vi "Initialize.vi"(8 "error in":errorcluster, 11 "Ballard ARINC-429 shared resources in":refnum<class "Ballard ARINC-429 Shared Resources.lvclass">) -> (0 "error out":errorcluster, 3 "Ballard ARINC-429 shared resources out":refnum<class "Ballard ARINC-429 Shared Resources.lvclass">)   [LabVIEW 2020, in "Ballard ARINC 429 Engine.lvlib" / "Implementation.lvlib" / "Ballard ARINC-429 Shared Resources.lvclass"]
uses:
  Ballard ARINC-429 Shared Resources.lvclass
  Ballard ARINC-429 Shared Resources.lvclass/Ballard ARINC-429 Shared Resources.ctl
  Custom Device/Custom Device.lvlib
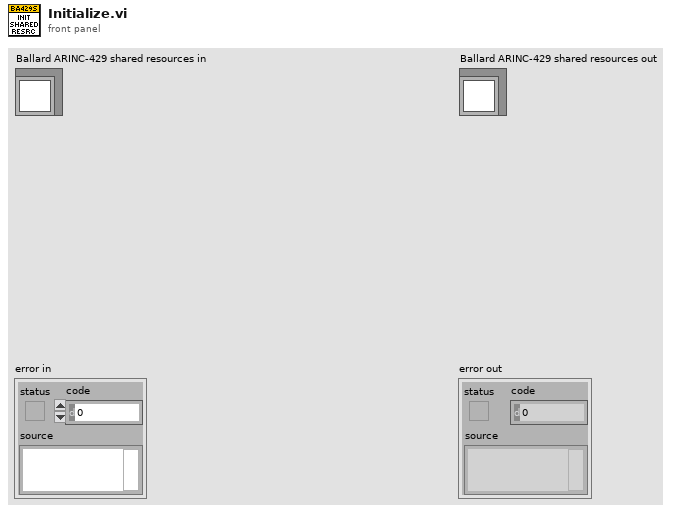
[diagram p1: front panel]
types:
  T1 = typedef "Device Parameters.ctl" = cluster{"initialization method":T2, "card number":i32, "PXI slot number":i32, "core number":i32}
  T2 = typedef "Initialization Method.ctl" = enum16{"PXI Slot Number", "Card Number"}
  T3 = typedef "Ballard ARINC 429 Engine.lvlib/Custom Device.lvlib/Hardware Handles.ctl" = cluster{"core handle":u64, "core reader handle":u64, "channel handles":u64[]}
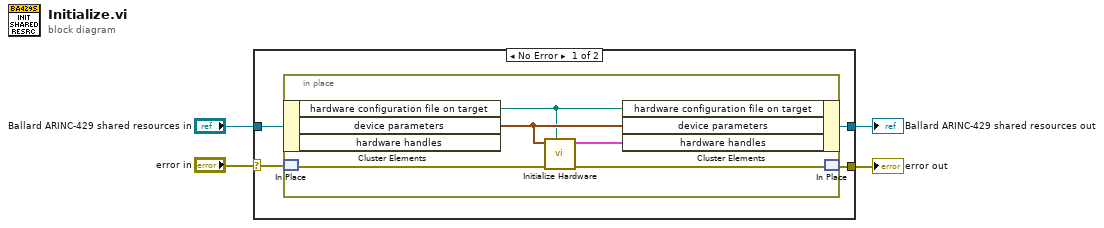
[diagram p0: block diagram]
diagram:
  n1 = case shown="No Error" "error in" {
    selector: "error in" -> [w8 w14]
    tunnel: "Ballard ARINC-429 shared resources in" -> [w6 w15]
    tunnel: [w7 w14] -> w2
    tunnel: [w5 w15] -> w1
    frame No Error {
      n2 = in-place {
        n3 = in-place-cluster #1(w6) -> ("hardware configuration file on target"=w9:path, "device parameters"=w10:T1)  [unwired: 1 out]
        n4 = in-place-match #2(w8) -> (w13:errorcluster)
        n5 = call "Initialize Hardware.vi"("RT config file"=w9, "error in"=w13, "device parameters"=w10) -> ("error out"=w12:errorcluster, "RT handles"=w11:T3)  [unwired: 6 in, 1 out]
        n6 = in-place-cluster #1("hardware configuration file on target"=w9, "device parameters"=w10, "hardware handles"=w11) -> (w5:refnum<class "Ballard ARINC-429 Shared Resources.lvclass">)
        n7 = in-place-match #2(w12) -> (w7:errorcluster)
      }
    }
    frame Error {
    }
  }
  "error out" <- w2
  "Ballard ARINC-429 shared resources out" <- w1
